vi "Get Array of LogicOut.vi"(8 "error in (no error)":errorcluster, 11 "VacuumLines Configuration in":refnum<class "VacuumLines Configuration.lvclass">) -> (0 "error out":errorcluster, 2 "Array of LogicOut":T1[](array[typedef]), 3 "VacuumLines Configuration out":refnum<class "VacuumLines Configuration.lvclass">)   [LabVIEW 2016, in "Hardware.lvlib" / "VacuumLine.lvlib" / "VacuumLines Configuration.lvclass"]
uses:
  <userlib>/Common Components/Hardware/Abstract System/VacuumLine/VacuumLines Configuration/VacuumLines Configuration.lvclass
  <userlib>/Common Components/Hardware/Abstract System/VacuumLine/VacuumLines/LogicOut.ctl
  <userlib>/Common Components/Hardware/Abstract System/VacuumLine/VacuumLines Configuration/VacuumLines Configuration.lvclass/VacuumLines Configuration.ctl
  <userlib>/Common Components/Hardware/Abstract System/VacuumLine/VacuumLines/VacuumLines.lvclass/VacuumLines.ctl
  <userlib>/Common Components/Hardware/Abstract System/VacuumLine/VacuumLines/VacuumLines.lvclass
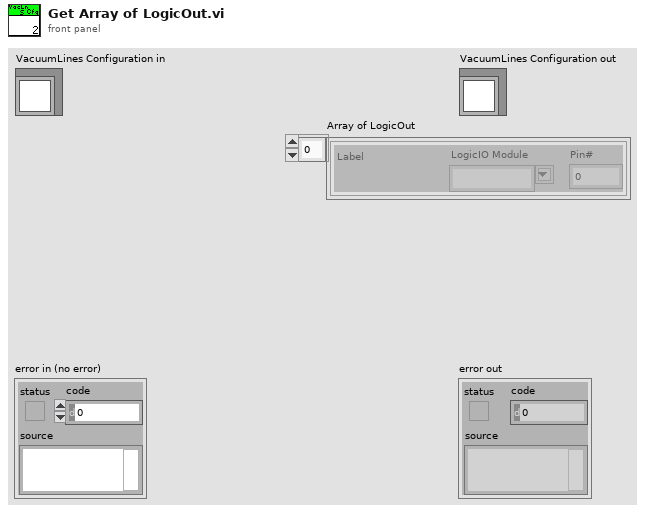
[diagram p1: front panel]
types:
  T1 = typedef "Hardware.lvlib/VacuumLine.lvlib/VacuumLines.lvclass/LogicOut.ctl" = cluster{"Label":string, "LogicIO Module":string, "Pin#":u8}
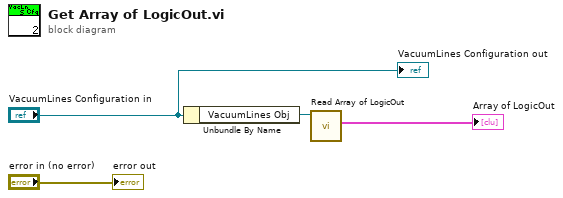
[diagram p0: block diagram]
diagram:
  n1 = Unbundle By Name("VacuumLines Configuration in") -> ("VacuumLines Obj"=w2:refnum<class "VacuumLines.lvclass">)
  n2 = call <userlib>:"Read Array of LogicOut.vi"("VacuumLines in"=w2) -> ("Array of LogicOut"=→"Array of LogicOut":T1[])  [unwired: 9 in, 1 out]
  "error out" <- "error in (no error)"
  "VacuumLines Configuration out" <- "VacuumLines Configuration in"
